vi "期末12.vi"() -> ()   [LabVIEW 2014]
uses:
  <vilib>/vision/NI_Vision_Development_Module.lvlib
panel:
  in  "3. Number of Erosion":i32=10
  in  "亮度控制":i64=128 min=0 max=255 step=1
  in  "紀錄":bool
  out "Image Out 2":T1(plugin-control)
  in  "紀錄中點座標和":bool
  out "Image Out":T1(plugin-control)
  in  "紀錄電流":dbl[](array[numeric])
  in  "Tab Control 2":enum32{"座標", "座標和", "作圖"}(tab)
  out "相減結果":dbl[](array[numeric])
  out "尖點座標和":dbl[](array[numeric])
  in  "計數器":dbl
  out "填入飽和磁場分量尖點座標和 2":dbl
  out "座標和":dbl
  out "分量-電流":cluster{"紀錄電流":dbl[], dbl[]}(graph)
  in  "結束實驗":bool
  in  "1. 範圍選擇":T2={"色相（H）"={0, 255}, "飽和度（S）"={0, 255}, "亮度（L）"={0, 255}} {"亮度（L）" scale=0.0..255.0; "飽和度（S）" scale=0.0..255.0; "色相（H）" scale=0.0..255.0}
  out "取點數":i32
  out "output cluster":cluster{"X":dbl, "Y":dbl}
  in  "Tab Control":T3(tab)
  out "1. 顏色選取":T1(plugin-control)
  out "2. 填補空隙":T1(plugin-control)
  out "3. 移除雜點":T1(plugin-control)
  out "4. 形狀修正":T1(plugin-control)
  out "5. 選取結果":T1(plugin-control)
  out "Particle Measurements":dbl[][](array[numeric])
  out "Error Out":errorcluster
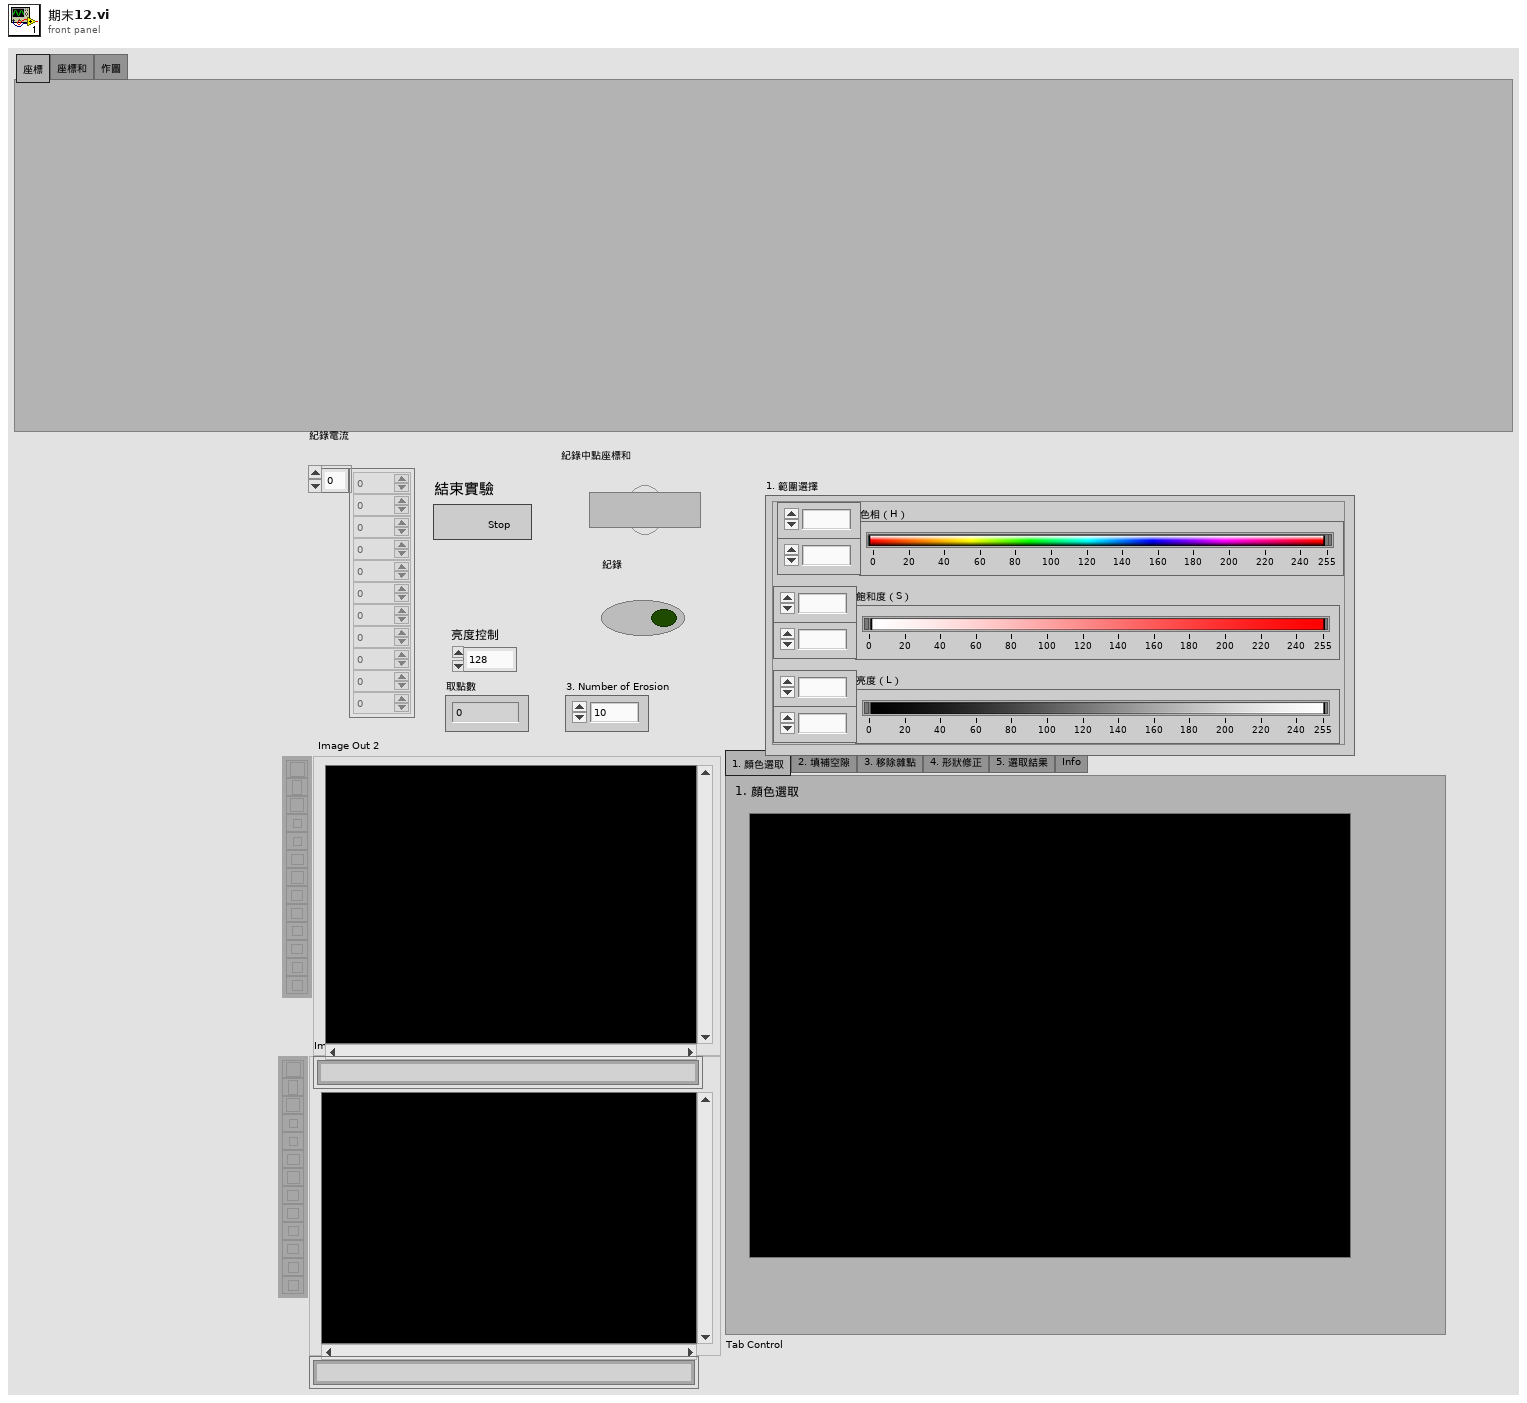
[diagram p1: front panel]
types:
  T1 = typedef "IMAQ Image.ctl" = refnum<image>
  T2 = cluster{"色相（H）":cluster{u8, u8}, "飽和度（S）":cluster{u8, u8}, "亮度（L）":cluster{u8, u8}}
  T3 = enum32{"1. 顏色選取", "2. 填補空隙", "3. 移除雜點", "4. 形狀修正", "5. 選取結果", "Info"}
  T4 = typedef "Image Type" = u32
  T5 = cluster{"Global Rectangle":i32[], "Contours":cluster{"Contour Type":u32, "ROI Type":u32, "Points":i32[]}[]}
  T6 = cluster{"Numeric":dbl, "Numeric":dbl, "Numeric":dbl, "Numeric":dbl}
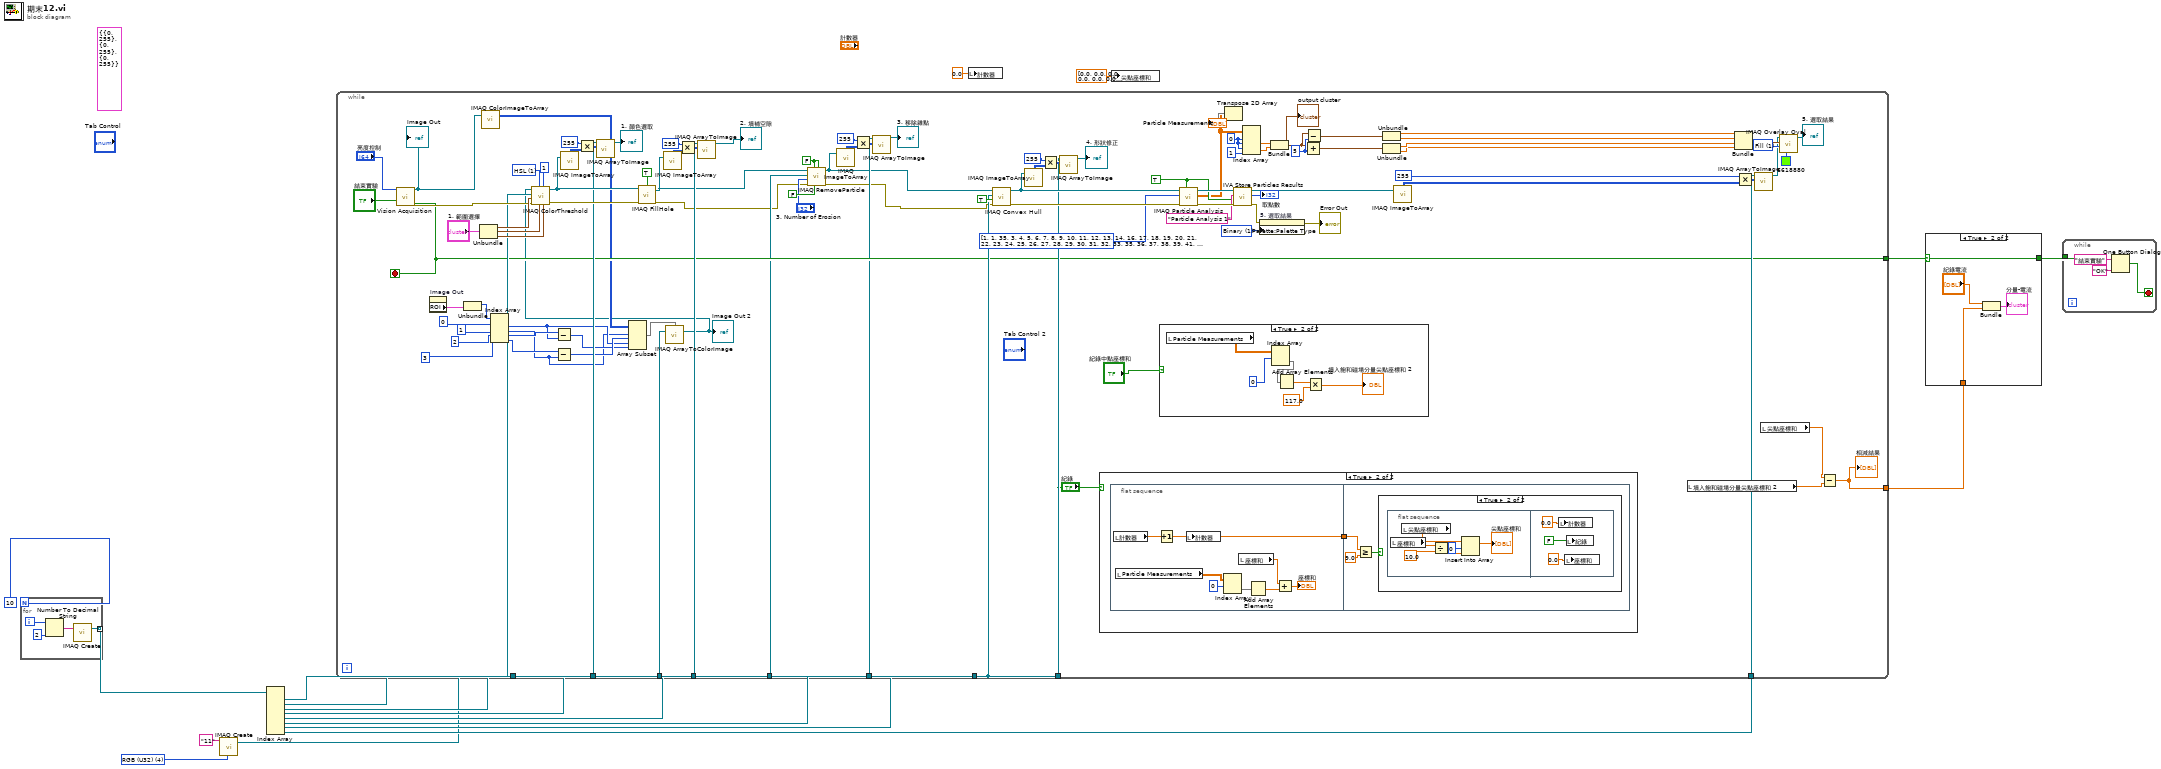
[diagram p0: block diagram]
diagram:
  w5 = T4 4 items=["Grayscale (U8)", "Grayscale (I16)", "Grayscale (SGL)", "Complex (CSG)", "RGB (U32)", "HSL (U32)", "RGB (U64)", "Grayscale (U16)"] ("Image Type")
  (unwired) T2 {"色相（H）"={0, 255}, "飽和度（S）"={0, 255}, "亮度（L）"={0, 255}} ("範圍選擇")
  n1 = for {
    N: 10 -> [_]
    tunnel: [w19] -> w18 mode=indexing
    i -> [w21]
    n2 = Number To Decimal String(number=w21, width (-)=2) -> (decimal integer string=w20:string)
    n3 = call "IMAQ Create"("Image Name"=w20) -> ("New Image"=w19:T1)  [unwired: 4 in, 1 out]
  }
  n4 = call "IMAQ Create"("Image Name"="11", "Image Type"=w5) -> ("New Image"=w6:T1)  [unwired: 3 in, 1 out]
  n5 = Index Array(array=w18) -> (element #1=w17:T1, element #2=w16:T1, element #3=w15:T1, element #4=w8:T1, element #5=w7:T1, element #6=w13:T1, element #7=w12:T1, element #8=w11:T1)  [unwired: 8 in]
  n6 = while {
    tunnel: w15 -> [w93]
    tunnel: w13 -> [w104]
    tunnel: [w104] -> _
    tunnel: w16 -> [w98]
    tunnel: w17 -> [w92]
    tunnel: w12 -> [w86]
    tunnel: w11 -> [w63]
    tunnel: [w59] -> w10
    tunnel: [w27] -> w9
    tunnel: w8 -> [w52]
    tunnel: w7 -> [w51]
    tunnel: w6 -> [w37]
    stop <- w59 stop-if-true
    w56 = FALSE ("Connectivity 4/8 (8)")
    w68 = u32 1 items=["Frame", "Fill"] ("Drawing Mode (Frame)")
    w77 = 5
    w82 = 0
    w106 = u32 1 items=["Grayscale", "Binary", "Gradient", "Rainbow", "Temperature", "User Defined"] ("Palette")
    w111 = i32[] [1, 1, 35, 3, 4, 5, 6, 7, 8, 9, 10, 11, 12, 13, 14, 16, 17, 18, 19, 20, 21, 22, 23, 24, 25, 26, 27, 28, 29, 30, 31, 32, 33, 35, 36, 37, 38, 39, 41, 42, 43, 45, 46, 48, 49, 50, 51, 53, 54, 55, 56, 58, 59, 60, 61, 62, 63, 64, 65, 66, 68, 69, 70, 71, 72, 73, 74, 75, 76, 77, 78, 79, 80, 81, 82, 83, 84, 85, 86, 87, 88] items=["Center of Mass X", "Center of Mass Y", "First Pixel X", "First Pixel Y", "Bounding Rect Left", "Bounding Rect Top", "Bounding Rect Right", "Bounding Rect Bottom", "Max Feret Diameter Start X", "Max Feret Diameter Start Y", "Max Feret Diameter End X", "Max Feret Diameter End Y", "Max Horiz. Segment Length Left", "Max Horiz. Segment Length Right", "Max Horiz. Segment Length Row", "-", "Bounding Rect Width", "Bounding Rect Height", "Bounding Rect Diagonal", "Perimeter", "Convex Hull Perimeter", "Holes' Perimeter", "Max Feret Diameter", "Equivalent Ellipse Major Axis", "Equivalent Ellipse Minor Axis", "Equivalent Ellipse Minor Axis (Feret)", "Equivalent Rect Long Side", "Equivalent Rect Short Side", "Equivalent Rect Diagonal", "Equivalent Rect Short Side (Feret)", "Average Horiz. Segment Length", "Average Vert. Segment Length", "Hydraulic Radius", "Waddel Disk Diameter", "-", "Area", "Holes' Area", "Particle & Holes' Area", "Convex Hull Area", "Image Area", "-", "Number of Holes", "Number of Horiz. Segments", "Number of Vert. Segments", "-", "Orientation", "Max Feret Diameter Orientation", "-", "% Area/Image Area", "% Area/(Particle & Holes' Area)", "Ratio of Equivalent Ellipse Axes", "Ratio of Equivalent Rect Sides", "-", "Elongation Factor", "Compactness Factor", "Heywood Circularity Factor", "Type Factor", "-", "Sum X", "Sum Y", "Sum XX", "Sum XY", "Sum YY", "Sum XXX", "Sum XXY", "Sum XYY", "Sum YYY", "-", "Moment of Inertia XX", "Moment of Inertia XY", "Moment of Inertia YY", "Moment of Inertia XXX", "Moment of Inertia XXY", "Moment of Inertia XYY", "Moment of Inertia YYY", "Norm. Moment of Inertia XX", "Norm. Moment of Inertia XY", "Norm. Moment of Inertia YY", "Norm. Moment of Inertia XXX", "Norm. Moment of Inertia XXY", "Norm. Moment of Inertia XYY", "Norm. Moment of Inertia YYY", "Hu Moment 1", "Hu Moment 2", "Hu Moment 3", "Hu Moment 4", "Hu Moment 5", "Hu Moment 6", "Hu Moment 7"] ("Pixel Measurements")
    w113 = TRUE ("Connectivity 4/8 (8)")
    w122 = u16 1 items=["RGB", "HSL", "HSV", "HSI"] ("Color Mode")
    n7 = call "Vision Acquisition"("Brightness::Value"="亮度控制", "Stop (F)"="結束實驗") -> ("Image Out"=w45:T1, "Stopped"=w59:bool, "error out"=w117:errorcluster)  [unwired: 23 in]
    "Image Out" <- w45
    n8 = property on="Image Out" class="ImageControl"() -> ("ROI"=w43:T5)  [unwired: 2 in, 2 out]
    n9 = Unbundle(w43) -> ("Global Rectangle"=w42:i32[])  [unwired: 1 out]
    n10 = Unbundle("1. 範圍選擇") -> ("色相（H）"=w121:cluster{u8, u8}, "飽和度（S）"=w120:cluster{u8, u8}, "亮度（L）"=w119:cluster{u8, u8})
    n11 = call "IMAQ ColorImageToArray"("Image"=w45) -> ("Image Pixels (U32)"=w44:u32[][])  [unwired: 3 in, 2 out]
    n12 = Index Array(array=w42, index #1=0 ("index"), index #2=1 ("index"), index #3=2 ("index"), index #4=3 ("index")) -> (element #1=w32:i32, element #2=w30:i32, element #3=w35:i32, element #4=w31:i32)
    n13 = Subtract(x=w35, y=w32) -> (x-y=w33:i32)
    n14 = Subtract(x=w31, y=w30) -> (x-y=w34:i32)
    n15 = Array Subset(array=w44, index (row)=w30, length (row)=w34, index (col)=w32, length (col)=w33) -> (w36:u32[][])
    n16 = call "IMAQ ArrayToColorImage"("Image Pixels (U32)"=w36, "Image"=w37) -> ("Image Out"=w29:T1)  [unwired: 3 in, 1 out]
    "Image Out 2" <- w29
    n17 = call "IMAQ ColorThreshold"("Blue or Luma or Val or Inten Range"=w119, "Replace Value"=1, "Green or Sat Range"=w120, "Color Mode"=w122, "error in (no error)"=w117, "Red or Hue Range"=w121, "Image Dst"=w92, "Image Src"=w29) -> ("error out"=w108:errorcluster, "Image Dst Out"=w103:T1)  [unwired: 2 out]
    n18 = call "IMAQ ImageToArray"("Image"=w103) -> ("Image Pixels (U8)"=w101:u8[][])  [unwired: 3 in, 4 out]
    n19 = Multiply(x=255, y=w101) -> (x*y=w100:i32[][])
    n20 = call "IMAQ ArrayToImage"("Image Pixels (U8)"=w100, "Image"=w98) -> ("Image Out"=→"1. 顏色選取":T1)  [unwired: 8 in, 1 out]
    n21 = call "IMAQ FillHole"("error in (no error)"=w108, "Image Src"=w103, "Connectivity 4/8 (8)"=TRUE) -> ("error out"=w50:errorcluster, "Image Dst Out"=w48:T1)  [unwired: 1 in, 2 out]
    n22 = call "IMAQ ImageToArray"("Image"=w48) -> ("Image Pixels (U8)"=w96:u8[][])  [unwired: 3 in, 4 out]
    n23 = Multiply(x=255, y=w96) -> (x*y=w97:i32[][])
    n24 = call "IMAQ ArrayToImage"("Image Pixels (U8)"=w97, "Image"=w93) -> ("Image Out"=→"2. 填補空隙":T1)  [unwired: 8 in, 1 out]
    n25 = call "IMAQ RemoveParticle"("Connectivity 4/8 (8)"=w56, "Low Pass/High Pass (Low)"=FALSE, "Square/Hexa (Square)"=w56, "error in (no error)"=w50, "Number of Erosion"="3. Number of Erosion", "Image Dst"=w52, "Image Src"=w48) -> ("error out"=w49:errorcluster, "Image Dst Out"=w47:T1)  [unwired: 3 out]
    n26 = call "IMAQ ImageToArray"("Image"=w47) -> ("Image Pixels (U8)"=w46:u8[][])  [unwired: 3 in, 4 out]
    n27 = Multiply(x=255, y=w46) -> (x*y=w54:i32[][])
    n28 = call "IMAQ ArrayToImage"("Image Pixels (U8)"=w54, "Image"=w51) -> ("Image Out"=→"3. 移除雜點":T1)  [unwired: 8 in, 1 out]
    n29 = call "IMAQ Convex Hull"("error in (no error)"=w49, "Connectivity 4/8 (8)"=TRUE, "Image Dst"=w104, "Image Src"=w47) -> ("error out"=w112:errorcluster, "Image Dst Out"=w87:T1)  [unwired: 6 out]
    n30 = call "IMAQ ImageToArray"("Image"=w87) -> ("Image Pixels (U8)"=w90:u8[][])  [unwired: 3 in, 4 out]
    n31 = Multiply(x=255, y=w90) -> (x*y=w91:i32[][])
    n32 = call "IMAQ ArrayToImage"("Image Pixels (U8)"=w91, "Image"=w86) -> ("Image Out"=→"4. 形狀修正":T1)  [unwired: 8 in, 1 out]
    n33 = case shown="True" "紀錄" {
      frame False {
      }
      frame True {
        n34 = flat-sequence {
          tunnel: [w126] -> w124
          tunnel: w124 -> [w133]
          frame #0 {
            n35 = local read "計數器"() -> (w126:dbl)
            n36 = local read "Particle Measurements"() -> (w125:dbl[][])
            n37 = Increment(x=w126) -> (x+1=w127:dbl)
            n38 = local write "計數器"(w127) -> ()
            n39 = Index Array(array=w125, index (row)=0) -> (element=w131:dbl[])  [unwired: 1 in]
            n40 = local read "座標和"() -> (w130:dbl)
            n41 = Add Array Elements(numeric array=w131) -> (sum=w128:dbl)
            n42 = Add(x=w130, y=w128) -> (x+y=→"座標和":dbl)
          }
          frame #1 {
            n43 = Greater Or Equal?(x=w133, y=9.0) -> (x >= y?=w135:bool)
            n44 = case shown="True" w135 {
              frame False {
              }
              frame True {
                n45 = flat-sequence {
                  frame #0 {
                    n46 = local read "座標和"() -> (w141:dbl)
                    n47 = local read "尖點座標和"() -> (w136:dbl[])
                    n48 = Divide(x=w141, y=10.0) -> (x/y=w139:dbl)
                    n49 = Insert Into Array(array=w136, index=0, new element=w139) -> (→"尖點座標和":dbl[])
                  }
                  frame #1 {
                    n50 = local write "計數器"(0.0 ("計數器")) -> ()
                    n51 = local write "座標和"(0.0 ("座標和")) -> ()
                    n52 = local write "紀錄"(FALSE ("Boolean")) -> ()
                  }
                }
              }
            }
          }
        }
      }
    }
    n53 = case shown="True" "紀錄中點座標和" {
      frame False {
      }
      frame True {
        n54 = local read "Particle Measurements"() -> (w149:dbl[][])
        n55 = Index Array(array=w149, index (row)=0) -> (element=w148:dbl[])  [unwired: 1 in]
        n56 = Add Array Elements(numeric array=w148) -> (sum=w147:dbl)
        n57 = Multiply(x=w147, y=117.0) -> (x*y=→"填入飽和磁場分量尖點座標和 2":dbl)
      }
    }
    n58 = call "IMAQ Particle Analysis"("Connectivity 4/8 (8)"=w113, "error in (no error)"=w112, "Pixel Measurements"=w111, "Image"=w87) -> ("error out"=w116:errorcluster, "Particle Measurements (Pixels)"=w83:dbl[][], "Image Out (duplicate)"=w114:T1)  [unwired: 1 in, 4 out]
    n59 = Transpose 2D Array(2D array=w83) -> (transposed array=→"Particle Measurements":dbl[][])
    n60 = call <vilib>:"IVA Store Particles Results.vi"("error in (no error)"=w116, "Connectivity 4/8 (8)"=w113, "Step Name"="Particle Analysis 1", "Image in"=w114) -> ("error out"=w107:errorcluster, "Number of Particles"=→"取點數":i32, "Image dup"=w67:T1)  [unwired: 5 out]
    n61 = Index Array(array=w83, index (row) #1=w82, index (col) #1=w82, index (row) #2=w82, index (col) #2=1) -> (element #1=w80:dbl, element #2=w79:dbl)
    n62 = property on="5. 選取結果" class="ImageControl"(error in=w107, "Palette:Palette Type"=w106) -> (error out=→"Error Out":errorcluster)  [unwired: 1 in, 1 out]
    n63 = Bundle("Numeric"=w80, "Numeric"=w79) -> (w76:cluster{"Numeric":dbl, "Numeric":dbl})  [unwired: 1 in]
    "output cluster" <- w76
    n64 = Add(x=w76, y=w77) -> (x+y=w74:cluster{"Numeric":dbl, "Numeric":dbl})
    n65 = Subtract(x=w76, y=w77) -> (x-y=w75:cluster{"Numeric":dbl, "Numeric":dbl})
    n66 = Unbundle(w75) -> ("Numeric"=w73:dbl, "Numeric"=w72:dbl)
    n67 = Unbundle(w74) -> ("Numeric"=w71:dbl, "Numeric"=w70:dbl)
    n68 = call "IMAQ ImageToArray"("Image"=w67) -> ("Image Pixels (U8)"=w64:u8[][])  [unwired: 3 in, 4 out]
    n69 = local read "填入飽和磁場分量尖點座標和 2"() -> (w28:dbl)
    n70 = Bundle("Numeric"=w73, "Numeric"=w72, "Numeric"=w71, "Numeric"=w70) -> (w69:T6)  [unwired: 1 in]
    n71 = Multiply(x=255, y=w64) -> (x*y=w65:i32[][])
    n72 = call "IMAQ ArrayToImage"("Image Pixels (U8)"=w65, "Image"=w63) -> ("Image Out"=w62:T1)  [unwired: 8 in, 1 out]
    n73 = local read "尖點座標和"() -> (w24:dbl[])
    n74 = call "IMAQ Overlay Oval"("Color"=u32 6618880, "Drawing Mode (Frame)"=w68, "Bounding Rectangle"=w69, "Image"=w62) -> ("Image Out"=→"5. 選取結果":T1)  [unwired: 6 in, 1 out]
    n75 = Subtract(x=w24, y=w28) -> (x-y=w27:dbl[])
    "相減結果" <- w27
  }
  n76 = local write "計數器"(0.0 ("計數器")) -> ()
  n77 = local write "尖點座標和"(dbl[] [0.0, 0.0, 0.0, 0.0, 0.0, 0.0, 0.0, 0.0, 0.0, 0.0, 0.0, 0.0, 0.0, 0.0, 0.0, 0.0, 0.0, 0.0, 0.0, 0.0, 0.0, 0.0, 0.0, 0.0, 0.0, 0.0, 0.0, 0.0, 0.0, 0.0, 0.0, 0.0, 0.0, 0.0, 0.0, 0.0, 0.0, 0.0, 0.0, 0.0, 0.0, 0.0, 0.0, 0.0, 0.0, 0.0, 0.0, 0.0, 0.0, 0.0, 0.0, 0.0, 0.0, 0.0, 0.0, 0.0, 0.0, 0.0, 0.0, 0.0, 0.0, 0.0, 0.0, 0.0, 0.0, 0.0, 0.0, 0.0, 0.0, 0.0, 0.0, 0.0, 0.0, 0.0, 0.0, 0.0, 0.0, 0.0, 0.0, 0.0, 0.0, 0.0, 0.0, 0.0, 0.0, 0.0, 0.0, 0.0, 0.0, 0.0, 0.0, 0.0, 0.0, 0.0, 0.0, 0.0, 0.0, 0.0, 0.0, 0.0, 0.0, 0.0, 0.0, 0.0, 0.0, 0.0, 0.0, 0.0, 0.0, 0.0, 0.0, 0.0, 0.0, 0.0, 0.0, 0.0, 0.0, 0.0, 0.0, 0.0, 0.0, 0.0, 0.0, 0.0, 0.0, 0.0, 0.0, 0.0, 0.0, 0.0, 0.0, 0.0, 0.0, 0.0, 0.0, 0.0, 0.0, 0.0, 0.0, 0.0, 0.0, 0.0, 0.0, 0.0, 0.0, 0.0, 0.0, 0.0, 0.0, 0.0, 0.0, 0.0, 0.0, 0.0, 0.0, 0.0, 0.0, 0.0, 0.0, 0.0, 0.0, 0.0, 0.0, 0.0, 0.0, 0.0, 0.0, 0.0, 0.0, 0.0, 0.0, 0.0, 0.0, 0.0, 0.0, 0.0, 0.0, 0.0, 0.0, 0.0, 0.0, 0.0, 0.0, 0.0, 0.0, 0.0, 0.0, 0.0, 0.0, 0.0, 0.0, 0.0, 0.0, 0.0, 0.0, 0.0, 0.0, 0.0, 0.0, 0.0, 0.0, 0.0, 0.0, 0.0, 0.0, 0.0, 0.0, 0.0, 0.0, 0.0, 0.0, 0.0, 0.0, 0.0, 0.0, 0.0, 0.0, 0.0, 0.0, 0.0, 0.0, 0.0, 0.0, 0.0, 0.0, 0.0, 0.0, 0.0, 0.0, 0.0, 0.0, 0.0, 0.0, 0.0, 0.0, 0.0, 0.0, 0.0, 0.0, 0.0, 0.0, 0.0, 0.0, 0.0, 0.0, 0.0, 0.0, 0.0, 0.0, 0.0, 0.0, 0.0, 0.0, 0.0, 0.0, 0.0, 0.0, 0.0, 0.0, 0.0, 0.0, 0.0, 0.0, 0.0, 0.0, 0.0, 0.0, 0.0, 0.0, 0.0, 0.0, 0.0, 0.0, 0.0, 0.0, 0.0, 0.0, 0.0, 0.0, 0.0, 0.0, 0.0, 0.0, 0.0, 0.0, 0.0, 0.0, 0.0, 0.0, 0.0, 0.0, 0.0, 0.0, 0.0, 0.0, 0.0, 0.0, 0.0, 0.0, 0.0, 0.0, 0.0, 0.0, 0.0, 0.0, 0.0, 0.0, 0.0, 0.0, 0.0, 0.0, 0.0, 0.0, 0.0, 0.0, 0.0, 0.0, 0.0, 0.0, 0.0, 0.0, 0.0, 0.0, 0.0, 0.0, 0.0, 0.0, 0.0, 0.0, 0.0, 0.0, 0.0, 0.0, 0.0, 0.0, 0.0, 0.0, 0.0, 0.0, 0.0, 0.0, 0.0, 0.0, 0.0, 0.0, 0.0, 0.0, 0.0, 0.0, 0.0, 0.0, 0.0, 0.0, 0.0, 0.0, 0.0, 0.0, 0.0, 0.0, 0.0, 0.0, 0.0, 0.0, 0.0, 0.0, 0.0, 0.0, 0.0, 0.0, 0.0, 0.0, 0.0, 0.0, 0.0, 0.0, 0.0, 0.0, 0.0, 0.0, 0.0, 0.0, 0.0, 0.0, 0.0, 0.0, 0.0, 0.0, 0.0, 0.0, 0.0, 0.0, 0.0, 0.0, 0.0, 0.0, 0.0, 0.0, 0.0, 0.0, 0.0, 0.0, 0.0, 0.0, 0.0, 0.0, 0.0, 0.0, 0.0, 0.0, 0.0, 0.0, 0.0, 0.0, 0.0, 0.0, 0.0, 0.0, 0.0, 0.0, 0.0, 0.0, 0.0, 0.0, 0.0, 0.0, 0.0, 0.0, 0.0, 0.0, 0.0, 0.0, 0.0, 0.0, 0.0, 0.0, 0.0, 0.0, 0.0, 0.0, 0.0, 0.0, 0.0, 0.0, 0.0, 0.0, 0.0, 0.0, 0.0, 0.0, 0.0, 0.0, 0.0, 0.0, 0.0, 0.0, 0.0, 0.0, 0.0, 0.0, 0.0, 0.0, 0.0, 0.0, 0.0, 0.0, 0.0, 0.0, 0.0, 0.0, 0.0, 0.0, 0.0, 0.0, 0.0, 0.0, 0.0, 0.0, 0.0, 0.0, 0.0, 0.0, 0.0, 0.0, 0.0, 0.0, 0.0, 0.0, 0.0, 0.0, 0.0, 0.0, 0.0, 0.0, 0.0, 0.0, 0.0, 0.0, 0.0, 0.0, 0.0, 0.0, 0.0, 0.0, 0.0, 0.0, 0.0, 0.0, 0.0, 0.0, 0.0, 0.0, 0.0, 0.0, 0.0, 0.0, 0.0, 0.0, 0.0, 0.0, 0.0, 0.0, 0.0, 0.0, 0.0, 0.0, 0.0, 0.0, 0.0, 0.0, 0.0, 0.0, 0.0, 0.0, 0.0, 0.0, 0.0, 0.0, 0.0, 0.0, 0.0, 0.0, 0.0, 0.0, 0.0, 0.0, 0.0, 0.0, 0.0, 0.0, 0.0, 0.0, 0.0, 0.0, 0.0, 0.0, 0.0, 0.0, 0.0, 0.0, 0.0, 0.0, 0.0, 0.0, 0.0, 0.0, 0.0, 0.0, 0.0, 0.0, 0.0, 0.0, 0.0, 0.0, 0.0, 0.0, 0.0, 0.0, 0.0, 0.0, 0.0, 0.0, 0.0, 0.0, 0.0, 0.0, 0.0, 0.0, 0.0, 0.0, 0.0, 0.0, 0.0, 0.0, 0.0, 0.0, 0.0, 0.0, 0.0, 0.0, 0.0, 0.0, 0.0, 0.0, 0.0, 0.0, 0.0, 0.0, 0.0, 0.0, 0.0, 0.0, 0.0, 0.0, 0.0, 0.0, 0.0, 0.0, 0.0, 0.0, 0.0, 0.0, 0.0, 0.0, 0.0, 0.0, 0.0, 0.0, 0.0, 0.0, 0.0, 0.0, 0.0, 0.0, 0.0, 0.0, 0.0, 0.0, 0.0, 0.0, 0.0, 0.0, 0.0, 0.0, 0.0, 0.0, 0.0, 0.0, 0.0, 0.0, 0.0, 0.0, 0.0, 0.0, 0.0, 0.0, 0.0, 0.0, 0.0, 0.0, 0.0, 0.0, 0.0, 0.0, 0.0, 0.0, 0.0, 0.0, 0.0, 0.0, 0.0] ("尖點座標和")) -> ()
  n78 = case shown="True" w10 {
    selector: w10 -> [w151 w155]
    tunnel: [w151 w155] -> w3
    tunnel: w9 -> [_ w154]
    frame False {
    }
    frame True {
      n79 = Bundle("紀錄電流"="紀錄電流", w154) -> (→"分量-電流":cluster{"紀錄電流":dbl[], dbl[]})  [unwired: 1 in]
    }
  }
  n80 = while {
    tunnel: w3 -> [_]
    stop <- w158 stop-if-true
    n81 = One Button Dialog(message="結束實驗", button name ("OK")="OK") -> (true=w158:bool)
  }
